vi "Get Data Analog In.vi"(7 "BufferSize":i32=512, 8 "error in (no error)":errorcluster, 9 "rgdSamples":dbl[](array[numeric]), 10 "idxChannel":i32, 11 "hdwf":i32) -> (0 "error out":errorcluster, 1 "rgdSamples out":dbl[](array[numeric]), 3 "function return":i32)   [LabVIEW 2012, in "AnalogDiscSDKLv.lvlib"]
doc: "extern \"C\" __declspec(dllexport) int GetData_AnalogIn(HDWF hdwf, \n int idxChannel, double rgdSamples[], int BufferSize );"
uses:
  <instrlib>/AnalogDiscSDKLv/AnalogDiscSDKLv.lvlib
  <instrlib>/AnalogDiscSDKLv/AnalogDiscSDKLv.dll
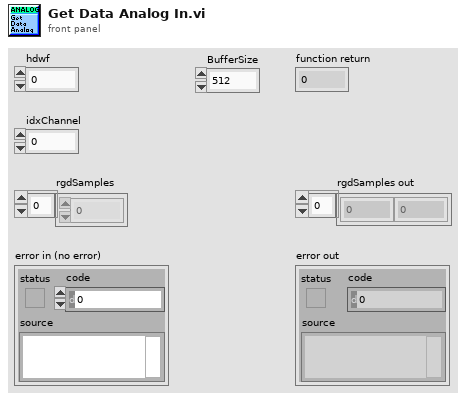
[diagram p1: front panel]
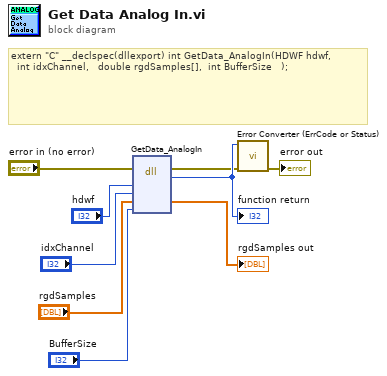
[diagram p0: block diagram]
diagram:
  # "extern \"C\" __declspec(dllexport) int GetData_AnalogIn(HDWF hdwf, \n\t\tint idxChannel,\t\t\tdouble rgdSamples[],\t\tint BufferSize\t\t\t);"
  n1 = dll-call lib="C:/Program Files (x86)/National Instruments/LabVIEW 2012/instr.lib/AnalogDiscSDKLv/AnalogDiscSDKLv.*" fn="GetData_AnalogIn"(error in="error in (no error)", "hdwf"="hdwf", "idxChannel"="idxChannel", "rgdSamples"="rgdSamples", "BufferSize"="BufferSize") -> (error out=w2:errorcluster, "return type"=w9:i32, "rgdSamples"=→"rgdSamples out":dbl[])  [unwired: 5 in, 1 out]
  "function return" <- w9
  n2 = call <instrlib>:"Error Converter (ErrCode or Status).vi"("error in (no error)"=w2, "error code"=w9) -> ("error out"=→"error out":errorcluster)  [unwired: 9 in]
